vi "Close Hardware Session.vi"(8 "error in":errorcluster, 11 "hardware handles":T1) -> (0 "error out":errorcluster)   [LabVIEW 2020, in "AIM MIL-STD-1553 Engine.lvlib" / "Custom Device.lvlib"]
uses:
  Custom Device.lvlib
  Hardware Handles.ctl
  <instrlib>/BTICardLib/BTICardLV.lvlib
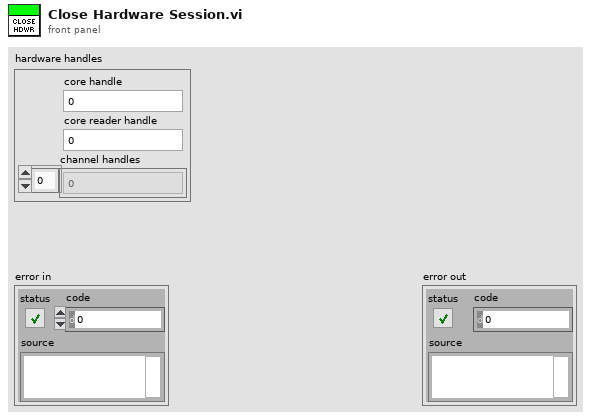
[diagram p1: front panel]
types:
  T1 = typedef "AIM MIL-STD-1553 Engine.lvlib/Custom Device.lvlib/Hardware Handles.ctl" = cluster{"core handle":u64, "core reader handle":u64, "channel handles":u64[]}
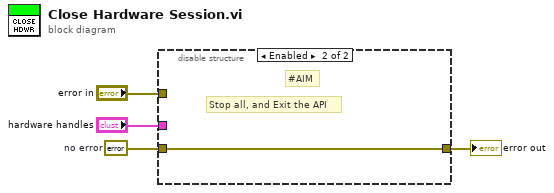
[diagram p0: block diagram]
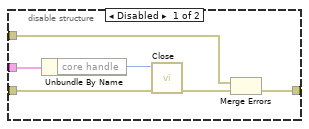
[diagram p2: hidden frame]
diagram:
  w1 = errorcluster {"status"=FALSE, "code"=0, "source"=""}  # no error
  n1 = disable-structure shown="Enabled" {
    disable-tunnel: "hardware handles" -> [w10 _]
    disable-tunnel: [w7 w11] -> w3
    disable-tunnel: "error in" -> [w6 _]
    disable-tunnel: w1 -> [w5 w11]
    frame Disabled {
      n2 = Unbundle By Name(w10) -> ("core handle"=w9:u64)
      n3 = call <instrlib>:"Close.vi"("error in (no error)"=w5, "core handle in"=w9) -> ("error out"=w8:errorcluster)  [unwired: 8 in, 1 out]
      n4 = Merge Errors(w6, w8) -> (w7:errorcluster)
    }
    frame Enabled {
      # "#AIM"
      # "Stop all, and Exit the API"
    }
  }
  "error out" <- w3
